vi "DCMotors Calibration.vi"() -> ()   [LabVIEW 2020]
uses:
  <vilib>/Platform/TimedLoop/XDataNode/timing_clust.ctl
  <vilib>/Platform/TimedLoop/XDataNode/nitl_modes.ctl
  <vilib>/Platform/TimedLoop/XDataNode/wakeup.ctl
  <vilib>/High Genius/HG_WSI_Tookit/Dependencies/Library/CAN/CAN.lvclass
  C:/Program Files (x86)/National Instruments/LabVIEW 2020/vi.lib/High Genius/HG_WSI_Tookit/Dependencies/Library/HG_LIB/HG_LIB.lvclass
  <vilib>/High Genius/HG_WSI_Tookit/Dependencies/Library/TitanENC/TitanENC.lvclass
  <vilib>/Platform/TimedLoop/XDataNode/XDataNode.xnode
  <vilib>/High Genius/HG_WSI_Tookit/Dependencies/Library/HG_LIB/HG_LIB.lvclass
panel:
  in  "Slide 3":dbl(slide)=0.5007832898172324 scale=0.4..0.6
  in  "Boolean 2":bool
  in  "Slide 2":dbl(slide) step=1.0 scale=-100.0..100.0
  in  "Input":dbl[](array[slide])=[0.0, 0.0, -0.01, 1.0] step=1.0 scale=-100.0..100.0
  out "Motors Renum Out":cluster{"Num":i32, "Directly":bool, "KM":dbl}[](array[cluster])=[{"Num"=0, "Directly"=TRUE, "KM"=1.0}, {"Num"=0, "Directly"=FALSE, "KM"=0.9987406674462534}, {"Num"=0, "Directly"=FALSE, "KM"=0.997932770088082}]
  in  "Reset Enc":bool
  in  "Slide":dbl(slide) step=1.0 scale=-100.0..100.0
  in  "Boolean":bool
  in  "Motors Renum":cluster{"Num":i32, "Directly":bool, "KM":dbl}[](array[cluster])=[{"Num"=1, "Directly"=TRUE, "KM"=1.0}, {"Num"=3, "Directly"=FALSE, "KM"=0.93}, {"Num"=0, "Directly"=FALSE, "KM"=0.95}]
  in  "Reset YAW":bool
  out "YAW (degree)":dbl
  out "ENC/dt":T1
  out "RPM":T2
  out "ENC True":T3
  out "ENC":T3
  out "error out":errorcluster
  in  "stop":bool
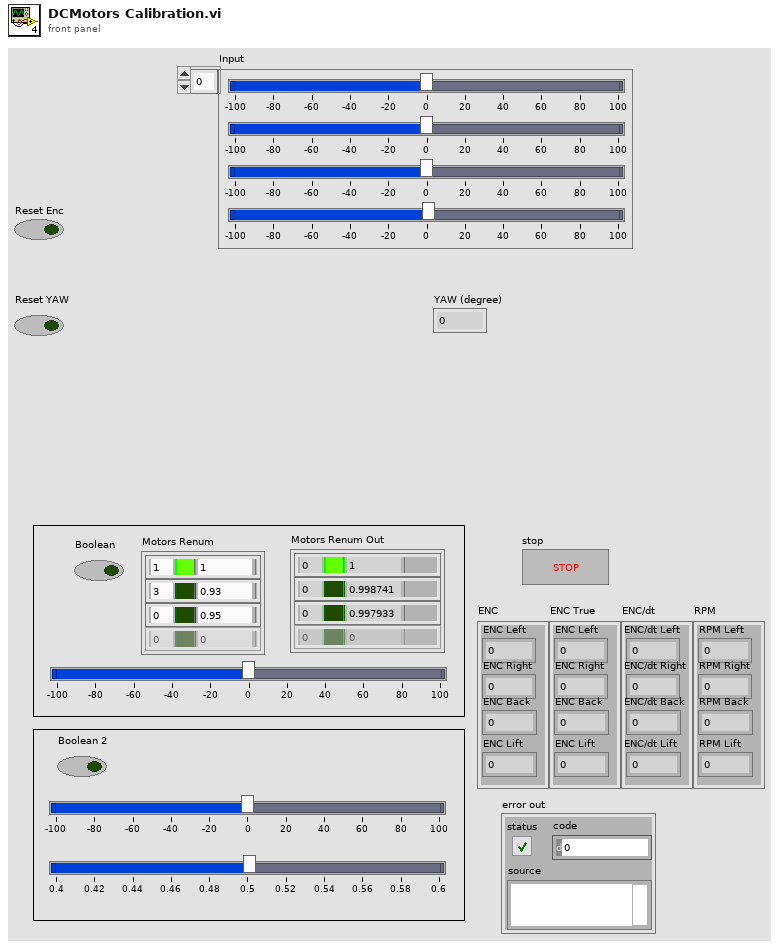
[diagram p1: front panel]
types:
  T1 = cluster{"ENC/dt Left":i32, "ENC/dt Right":i32, "ENC/dt Back":i32, "ENC/dt Lift":i32}
  T2 = cluster{"RPM Left":i32, "RPM Right":i32, "RPM Back":i32, "RPM Lift":i32}
  T3 = cluster{"ENC Left":i32, "ENC Right":i32, "ENC Back":i32, "ENC Lift":i32}
  T4 = cluster{"TitanENC 0":refnum<class "TitanENC.lvclass">, "TitanENC 1":refnum<class "TitanENC.lvclass">, "TitanENC 2":refnum<class "TitanENC.lvclass">, "TitanENC 3":refnum<class "TitanENC.lvclass">}
  T5 = typedef "XDNodeRunTimeDep.lvlib/timing_clust.ctl" = cluster{"Expected End [f-1]":u64, "Actual End [f-1]":u64, "Finished Late? [f-1]":bool, "Expected End [i-1]":u64, "Actual End [i-1]":u64, "Finished Late? [i-1]":bool, "Expected Start [i]":u64, "Actual Start [i]":u64, "Expected Start [f]":u64, "Actual Start [f]":u64, "Source Name":string, "Structure Name":string, "Period":i64, "Deadline":i64, "Offset":i64, "Start":i64, "Priority":i32, "Timeout":i32, "Mode":T6, "Wakeup Reason":T7, "Error":errorcluster, "Source Type":string, "Secondary Source Type":string, "Global End Time":u64, "Global Start Time":u64, "Frame Duration":u64, "Iteration Duration":u64, "Assigned CPU":i32, "I/O Scan Engine Mode":u32}
  T6 = typedef "XDNodeRunTimeDep.lvlib/nitl_modes.ctl" = enum32{"No Change", "Process missed periods, maintain original phase", "Discard missed periods, maintain original phase", "Process missed periods, ignore original phase", "Discard missed periods, ignore original phase"}
  T7 = typedef "XDNodeRunTimeDep.lvlib/wakeup.ctl" = enum32{"Normal", "Aborted", "Asynchronous wakeup", "Timing source error", "Timed loop error", "Timeout"}
  T8 = cluster{"TitanENC out":refnum<class "TitanENC.lvclass">, "TitanENC out":refnum<class "TitanENC.lvclass">, "TitanENC out":refnum<class "TitanENC.lvclass">, "TitanENC out":refnum<class "TitanENC.lvclass">}
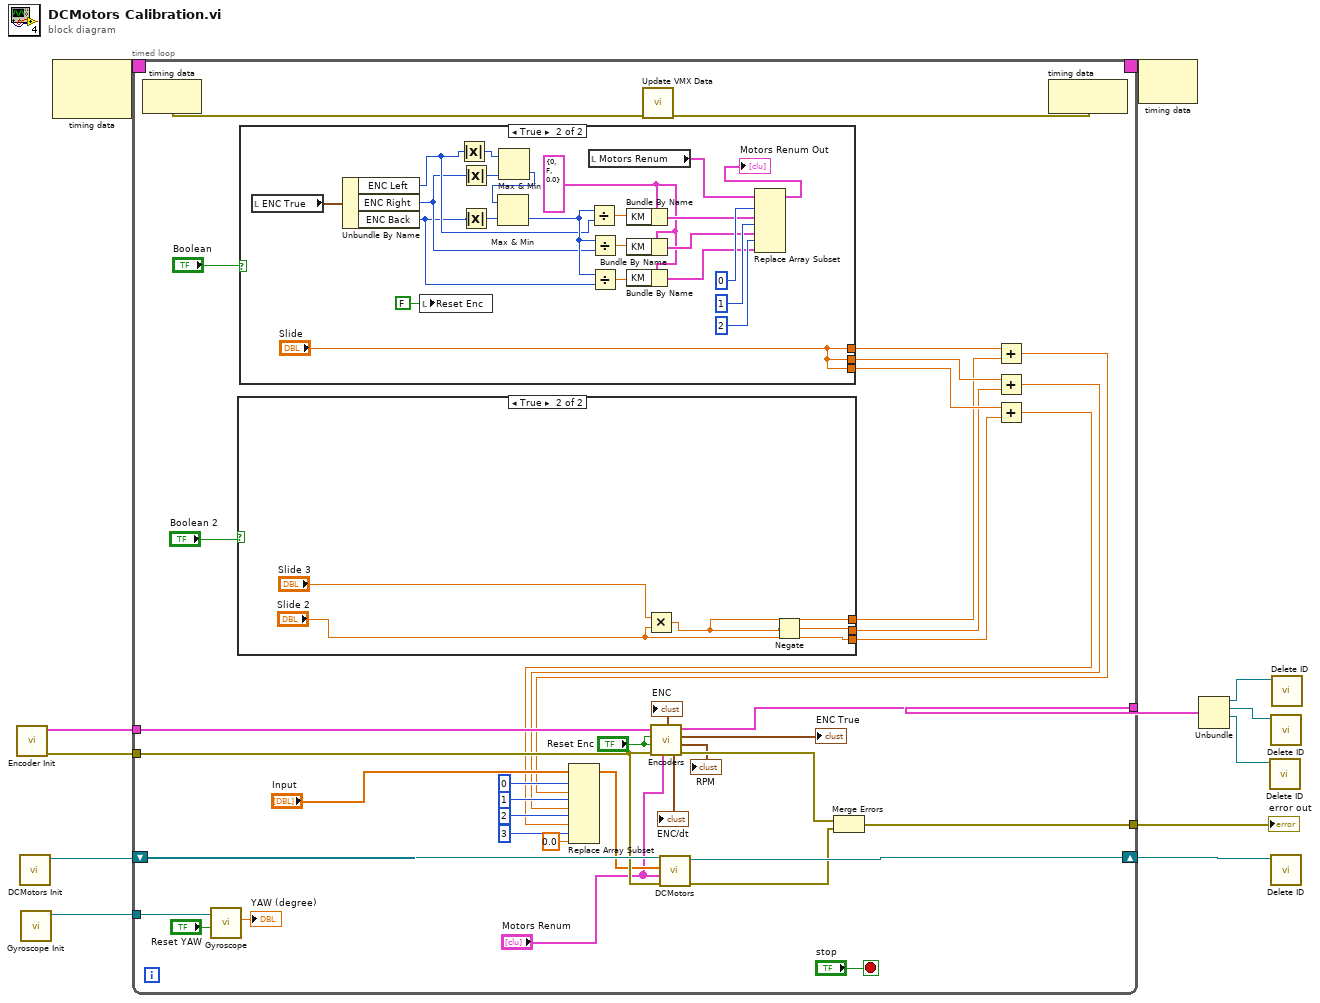
[diagram p0: block diagram]
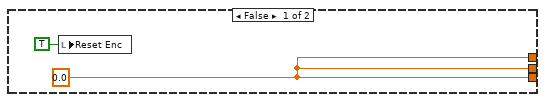
[diagram p2: hidden frame]
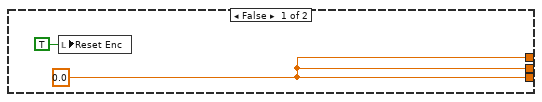
[diagram p3: hidden frame]
diagram:
  n1 = call "Encoder Init.vi"() -> ("error out"=w3:errorcluster, "TitanENC out"=w4:T4)  [unwired: 10 in]
  n2 = call "DCMotors Init.vi"() -> ("DC Motors"=w2:refnum<class "CAN.lvclass">)  [unwired: 10 in, 1 out]
  n3 = call "Gyroscope Init.vi"() -> ("Gyroscope"=w1:refnum<class "IMU.lvclass">)  [unwired: 10 in, 1 out]
  n4 = node-c288() -> (w12:T5)  [unwired: 2 in]
  n5 = timed-loop {
    timing: w12 -> [_]
    timing-out: [_] -> w11
    shift-right: [w49] -> w10
    shift-left: w2 -> [w50]
    tunnel: w3 -> [w44]
    tunnel: w4 -> [w45]
    tunnel: [w43] -> w9
    tunnel: [w40] -> w6
    tunnel: w1 -> [w31]
    stop <- "stop" stop-if-true
    n6 = node-c288() -> (w48:errorcluster)  [unwired: 1 in]
    n7 = call "Gyroscope.vi"("Reset YAW"="Reset YAW", "IMU in"=w31) -> ("YAW (degree)"=→"YAW (degree)":dbl)  [unwired: 5 in, 4 out]
    n8 = case shown="True" "Boolean 2" {
      tunnel: [w51 w53] -> w13
      tunnel: [w51 w54] -> w14
      tunnel: [w51 "Slide 2"] -> w15
      frame False {
        w51 = 0.0 ("Slide")
        n9 = local write "Reset Enc"(TRUE ("Reset Enc")) -> ()
      }
      frame True {
        n10 = Multiply(x="Slide 3", y="Slide 2") -> (x*y=w53:dbl)
        n11 = Negate(x=w53) -> (-x=w54:dbl)
      }
    }
    n12 = case shown="True" "Boolean" {
      tunnel: [w57 "Slide"] -> w22
      tunnel: [w57 "Slide"] -> w21
      tunnel: [w57 "Slide"] -> w20
      frame False {
        w57 = 0.0 ("Slide")
        n13 = local write "Reset Enc"(TRUE ("Reset Enc")) -> ()
      }
      frame True {
        w71 = cluster{"Num":i32, "Directly":bool, "KM":dbl} {"Num"=0, "Directly"=FALSE, "KM"=0.0} ("new element/subarray")
        n14 = local read "ENC True"() -> (w80:T3)
        n15 = Unbundle By Name(w80) -> ("ENC Left"=w62:i32, "ENC Right"=w61:i32, "ENC Back"=w60:i32)
        n16 = local write "Reset Enc"(FALSE ("Reset Enc")) -> ()
        n17 = Absolute Value(x=w62) -> (abs(x)=w67:i32)
        n18 = Absolute Value(x=w61) -> (abs(x)=w66:i32)
        n19 = Absolute Value(x=w60) -> (abs(x)=w65:i32)
        n20 = Max & Min(x=w67, y=w66) -> (min(x,y)=w64:i32)  [unwired: 1 out]
        n21 = Max & Min(x=w64, y=w65) -> (min(x,y)=w63:i32)  [unwired: 1 out]
        n22 = local read "Motors Renum"() -> (w79:cluster{"Num":i32, "Directly":bool, "KM":dbl}[])
        n23 = Divide(x=w63, y=w62) -> (x/y=w70:dbl)
        n24 = Divide(x=w63, y=w61) -> (x/y=w69:dbl)
        n25 = Divide(x=w63, y=w60) -> (x/y=w68:dbl)
        n26 = Bundle By Name(cluster=w71, "KM"=w70) -> (w74:cluster{"Num":i32, "Directly":bool, "KM":dbl})
        n27 = Bundle By Name(cluster=w71, "KM"=w69) -> (w73:cluster{"Num":i32, "Directly":bool, "KM":dbl})
        n28 = Bundle By Name(cluster=w71, "KM"=w68) -> (w72:cluster{"Num":i32, "Directly":bool, "KM":dbl})
        n29 = Replace Array Subset(array=w79, new element #1=w74, index #1=0 ("index"), new element #2=w73, index #2=1 ("index"), new element #3=w72, index #3=2 ("index")) -> (→"Motors Renum Out":cluster{"Num":i32, "Directly":bool, "KM":dbl}[])
      }
    }
    n30 = call <vilib>:"Update VMX Data.vi"("error in (no error)"=w48) -> ("error out"=w47:errorcluster)  [unwired: 10 in]
    n31 = call "Encoders.vi"("Motors Renum"="Motors Renum", "error in (no error)"=w44, "Reset Enc"="Reset Enc", "Start"="Reset Enc", "TitanENC in"=w45) -> ("error out"=w42:errorcluster, "RPM"=→"RPM":T2, "ENC True"=→"ENC True":T3, "TitanENC out"=w43:T8, "ENC/dt"=→"ENC/dt":T1, "ENC"=→"ENC":T3)  [unwired: 1 in]
    n32 = Add(x=w22, y=w13) -> (x+y=w19:dbl)
    n33 = Add(x=w21, y=w14) -> (x+y=w18:dbl)
    n34 = Add(x=w20, y=w15) -> (x+y=w17:dbl)
    n35 = Replace Array Subset(array="Input", new element #1=w19, index #1=0 ("index"), new element #2=w18, index #2=1 ("index"), new element #3=w17, index #3=2 ("index"), new element #4=0.0 ("new element/subarray"), index #4=3 ("index")) -> (w27:dbl[])
    n36 = call "DCMotors.vi"("error in"=w44, "Motors Renum"="Motors Renum", "Input"=w27, "CAN in"=w50) -> ("error out"=w41:errorcluster, "CAN out"=w49:refnum<class "CAN.lvclass">)  [unwired: 6 in]
    n37 = Merge Errors(w42, w41) -> (w40:errorcluster)
    n38 = node-c288(w47) -> ()  [unwired: 1 out]
  }
  "error out" <- w6
  n39 = node-c288(w11) -> ()  [unwired: 1 out]
  n40 = Unbundle(w9) -> ("TitanENC out"=w8:refnum<class "TitanENC.lvclass">, "TitanENC out"=w5:refnum<class "TitanENC.lvclass">, "TitanENC out"=w7:refnum<class "TitanENC.lvclass">)  [unwired: 1 out]
  n41 = call <vilib>:"Delete ID.vi"("HG_LIB in"=w7) -> ()  [unwired: 9 in, 2 out]
  n42 = call <vilib>:"Delete ID.vi"("HG_LIB in"=w5) -> ()  [unwired: 9 in, 2 out]
  n43 = call <vilib>:"Delete ID.vi"("HG_LIB in"=w10) -> ()  [unwired: 9 in, 2 out]
  n44 = call <vilib>:"Delete ID.vi"("HG_LIB in"=w8) -> ()  [unwired: 9 in, 2 out]
